vi "get log.vi"(7 "rw":T1, 8 "error in (no error)":errorcluster caption="에러 입력(에러 없음)", 9 "data":u8[](array[numeric]), 10 "start addr":u32, 11 "I2C 입력":refnum<class "I2C.lvclass">) -> (0 "error out":errorcluster caption="에러 출력", 2 "log_multiple line":string[](array[string]), 3 "I2C 출력":refnum<class "I2C.lvclass">, 4 "log_single line":string)   [LabVIEW 2020, in "I2C.lvclass"]
uses:
  I2C.lvclass
  Controls/(Ctrl)log & script_rw enum.ctl
  Controls/(Ctrl)i2c slv addr format fgv enum.ctl
  I2C.lvclass/I2C.ctl
  Accessors/Read address byte.vi
  Accessors/Read data byte.vi
  Accessors/Read slave address.vi
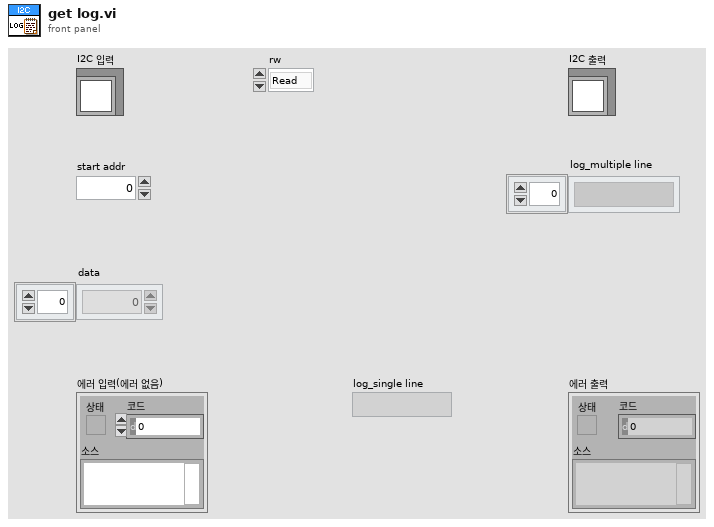
[diagram p1: front panel]
types:
  T1 = typedef "I2C.lvclass/(Ctrl)log & script_rw enum.ctl" = enum16{"Read", "Write"}
  T2 = typedef "I2C.lvclass/(Ctrl)i2c slv addr format fgv enum.ctl" = enum16{"Read", "Write"}
  T3 = typedef "I2C.lvclass/(Ctrl)i2c slv addr format.ctl" = enum16{"7bit", "8bit"}
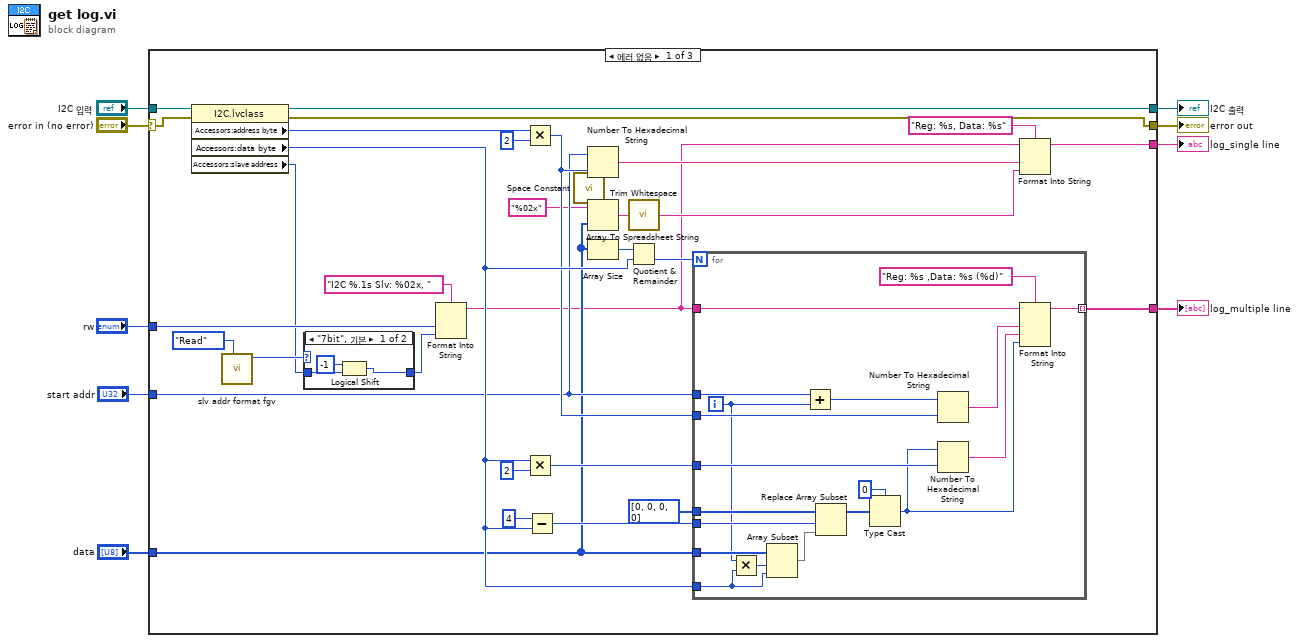
[diagram p0: block diagram]
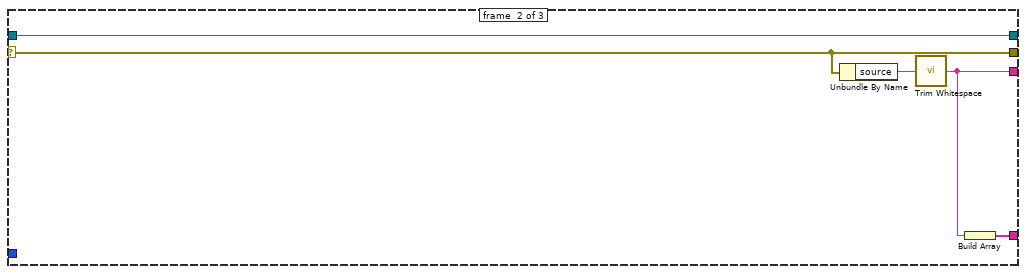
[diagram p3: hidden frame]
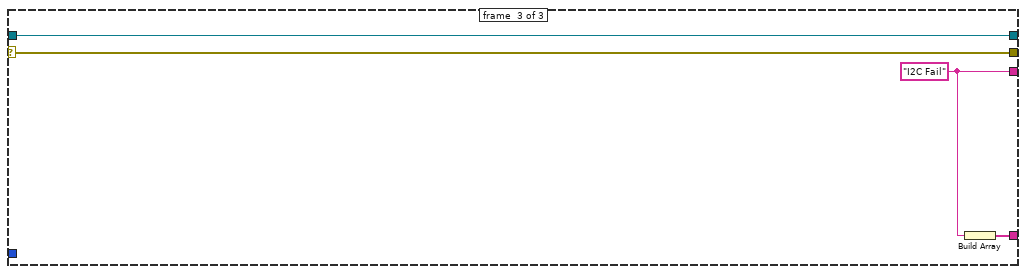
[diagram p4: hidden frame]
diagram:
  n1 = case shown="에러 없음" "error in (no error)" {
    selector: "error in (no error)" -> [w38 w68 w72]
    tunnel: [w37 w68 w72] -> w8
    tunnel: [w40 w69 w73] -> w6
    tunnel: "I2C 입력" -> [w41 w69 w73]
    tunnel: "rw" -> [w36 _ _]
    tunnel: "start addr" -> [w18 _ _]
    tunnel: "data" -> [w16 _ _]
    tunnel: [w33 w66 w71] -> w2
    tunnel: [w11 w65 w70] -> w1
    frame #0 {
      n2 = property class="I2C.lvclass"(reference=w41, error in=w38) -> (reference out=w40:refnum<class "I2C.lvclass">, error out=w37:errorcluster, "Accessors:address byte"=w35:u8, "Accessors:data byte"=w34:u8, "Accessors:slave address"=w30:u8)
      n3 = call "slv addr format fgv.vi"("function"=(Ctrl)i2c_slv_addr_format_fgv_enum."Read") -> ("i2c slv addr format out"=w31:T3)  [unwired: 9 in, 1 out]
      n4 = case shown="\"7bit\", 기본" w31 {
        tunnel: w30 -> [w63 w64]
        tunnel: [w61 w64] -> w29
        frame "7bit", Default {
          n5 = Logical Shift(y=i16 -1, x=w63) -> (x << y=w61:u8)
        }
        frame "8bit" {
        }
      }
      n6 = Format Into String(format string="I2C %.1s Slv: %02x, " ("포맷 문자열"), w36, w29) -> (resulting string=w10:string)  [unwired: 2 in, 1 out]
      n7 = Multiply(x=w35, y=u8 2) -> (x*y=w19:u8)
      n8 = Multiply(x=w34, y=u8 2) -> (x*y=w21:u8)
      n9 = Subtract(x=u8 4, y=w34) -> (x-y=w24:u8)
      n10 = call <vilib>:"Space Constant.vi"() -> ("String"=w14:string)
      n11 = Number To Hexadecimal String(1:w19, 2:w18) -> (0:w17:string)
      n12 = Array To Spreadsheet String(delimiter (Tab)=w14, array=w16, 3:"%02x" ("포맷 문자열")) -> (spreadsheet string=w13:string)
      n13 = Array Size(array=w16) -> (size(s)=w28:i32)
      n14 = call <vilib>:"Trim Whitespace.vi"("string"=w13) -> ("trimmed string"=w12:string)  [unwired: 1 in]
      n15 = Quotient & Remainder(x=w28, y=w34) -> (floor(x/y)=w27:i32)  [unwired: 1 out]
      n16 = for {
        N: w27 -> [_]
        tunnel: w18 -> [w60]
        tunnel: w34 -> [w50]
        tunnel: w16 -> [w52]
        tunnel: w10 -> [w59]
        tunnel: [w55] -> w33 mode=indexing
        tunnel: u8[] [0, 0, 0, 0] ("원소") -> [w54]
        tunnel: w24 -> [w53]
        tunnel: w19 -> [w44]
        tunnel: w21 -> [w46]
        i -> [w42]
        n17 = Multiply(x=w42, y=w50) -> (x*y=w51:i32)
        n18 = Array Subset(array=w52, index=w51, length=w50) -> (w49:u8[])
        n19 = Add(x=w60, y=w42) -> (x+y=w43:u32)
        n20 = Replace Array Subset(array=w54, new element=w49, index=w53) -> (w48:u8[])
        n21 = Type Cast(type=u32 0 ("타입"), x=w48) -> (*(type *) &x=w45:u32)
        n22 = Number To Hexadecimal String(1:w44, 2:w43) -> (0:w57:string)
        n23 = Number To Hexadecimal String(1:w46, 2:w45) -> (0:w56:string)
        n24 = Format Into String(format string="Reg: %s ,Data: %s (%d)" ("포맷 문자열"), initial string=w59, w57, w56, w45) -> (resulting string=w55:string)  [unwired: 1 in, 1 out]
      }
      n25 = Format Into String(format string="Reg: %s, Data: %s" ("포맷 문자열"), initial string=w10, w17, w12) -> (resulting string=w11:string)  [unwired: 1 in, 1 out]
    }
    frame #1 {
      n26 = Unbundle By Name(w68) -> ("source"=w67:string)
      n27 = call <vilib>:"Trim Whitespace.vi"("string"=w67) -> ("trimmed string"=w65:string)  [unwired: 1 in]
      n28 = Build Array(w65) -> (w66:string[])
    }
    frame #2 {
      w70 = "I2C Fail" ("source")
      n29 = Build Array(w70) -> (w71:string[])
    }
  }
  "error out" <- w8
  "I2C 출력" <- w6
  "log_multiple line" <- w2
  "log_single line" <- w1
